vi "Test Reshape Array.vi"() -> ()   [LabVIEW 2014]
panel:
  out "output array":i32[][](array[numeric])
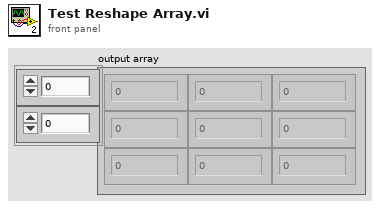
[diagram p1: front panel]
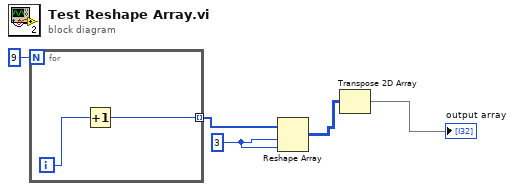
[diagram p0: block diagram]
diagram:
  w3 = 3 ("dimension size")
  n1 = for {
    N: 9 -> [_]
    tunnel: [w6] -> w4 mode=indexing
    i -> [w7]
    n2 = Increment(x=w7) -> (x+1=w6:i32)
  }
  n3 = Reshape Array(w4, w3, w3) -> (w2:i32[][])
  n4 = Transpose 2D Array(2D array=w2) -> (transposed array=→"output array":i32[][])
